vi "dataqsdk2008.vi"() -> ()   [LabVIEW 2019]
panel:
  out "Chan2":dbl(slide) scale=0.0..100.0
  out "Chan1":dbl(slide) scale=0.0..100.0
  in  "SampleRate":dbl=10.0
  in  "DeviceDriver":string="DI350NT.DLL"
  out "Two K-type inputs":dbl[][](graph)
  out "Channel 2 (K type)":dbl(knob) scale=-200.0..1372.0
  out "Channel 1 (K type)":dbl(knob) scale=-200.0..1372.0
  in  "DataqSdk":refnum<k7>(container)
  in  "Start/Stop":bool
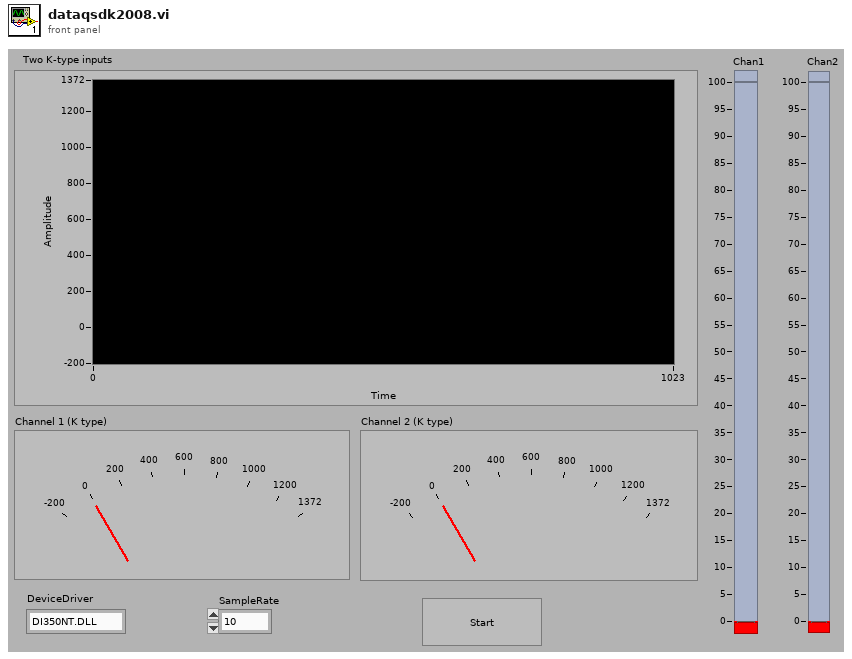
[diagram p1: front panel]
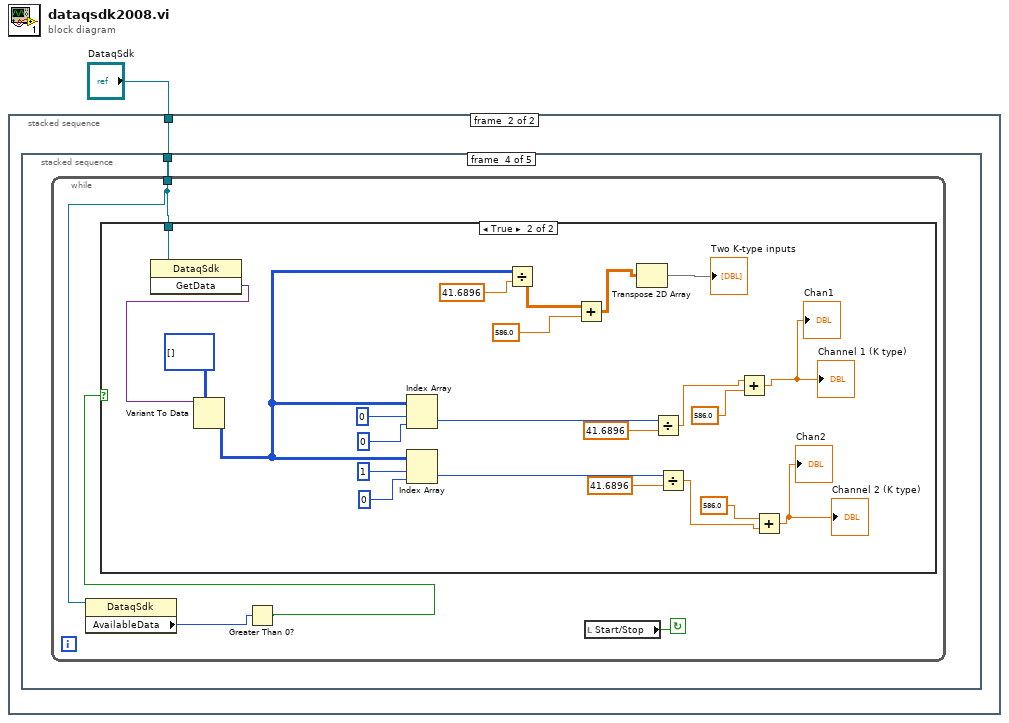
[diagram p0: block diagram]
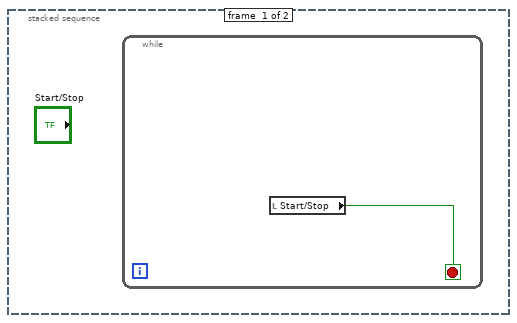
[diagram p2: hidden frame]
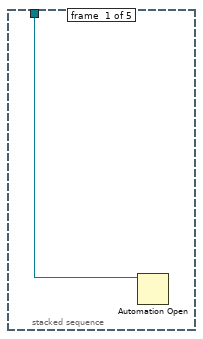
[diagram p3: hidden frame]
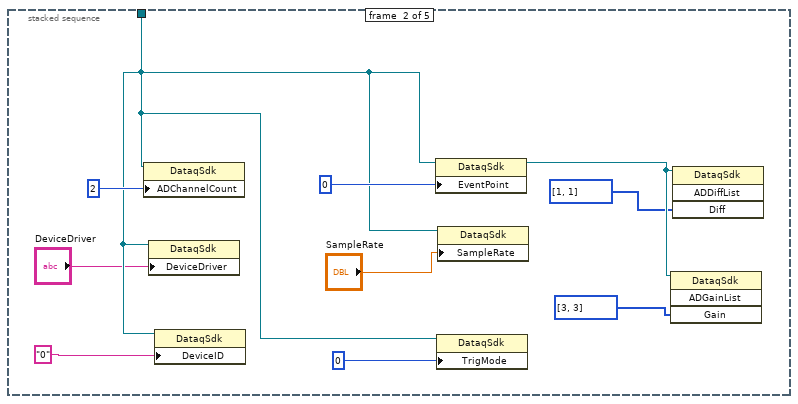
[diagram p4: hidden frame]
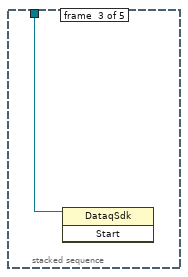
[diagram p5: hidden frame]
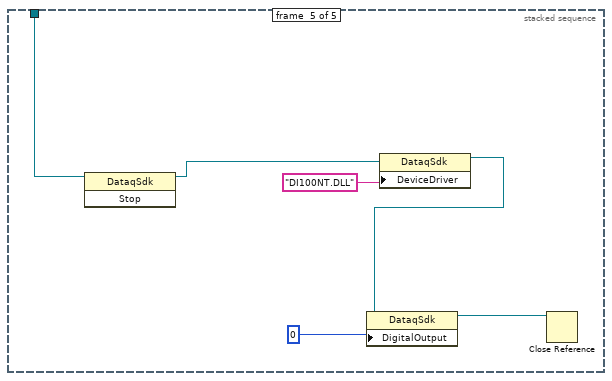
[diagram p7: hidden frame]
diagram:
  n1 = stacked-sequence {
    tunnel: "DataqSdk" -> [_ w3]
    frame #0 {
      n2 = while {
        stop <- w2 stop-if-true
        n3 = local read "Start/Stop"() -> (w2:bool)
      }
    }
    frame #1 {
      n4 = stacked-sequence {
        tunnel: w3 -> [w4 w12 w15 w16 w49]
        frame #0 {
          n5 = Automation Open(Automation Refnum=w4) -> ()  [unwired: 3 in, 2 out]
        }
        frame #1 {
          n6 = property class="DataqSdk"(reference=w12, "ADChannelCount"=2) -> ()  [unwired: 1 in, 2 out]
          n7 = property class="DataqSdk"(reference=w12, "DeviceDriver"="DeviceDriver") -> ()  [unwired: 1 in, 2 out]
          n8 = property class="DataqSdk"(reference=w12, "DeviceID"="0") -> ()  [unwired: 1 in, 2 out]
          n9 = property class="DataqSdk"(reference=w12, "EventPoint"=0) -> (reference out=w7:refnum<k7>)  [unwired: 1 in, 1 out]
          n10 = property class="DataqSdk"(reference=w12, "TrigMode"=0) -> ()  [unwired: 1 in, 2 out]
          n11 = property class="DataqSdk"(reference=w12, "SampleRate"="SampleRate") -> ()  [unwired: 1 in, 2 out]
          n12 = invoke class="DataqSdk" method="ADGainList"(reference=w7, "Gain"=i32[] [3, 3] ("Array")) -> ()  [unwired: 2 in, 4 out]
          n13 = invoke class="DataqSdk" method="ADDiffList"(reference=w7, "Diff"=i32[] [1, 1] ("Array")) -> ()  [unwired: 2 in, 4 out]
        }
        frame #2 {
          n14 = invoke class="DataqSdk" method="Start"(reference=w15) -> ()  [unwired: 2 in, 3 out]
        }
        frame #3 {
          n15 = while {
            tunnel: w16 -> [w19]
            stop <- w20 continue-if-true
            n16 = property class="DataqSdk"(reference=w19) -> ("AvailableData"=w18:i32)  [unwired: 1 in, 2 out]
            n17 = Greater Than 0?(x=w18) -> (x > 0?=w17:bool)
            n18 = case shown="True" w17 {
              tunnel: w19 -> [_ w43]
              frame False {
              }
              frame True {
                n19 = invoke class="DataqSdk" method="GetData"(reference=w43) -> ("GetData"=w39:variant)  [unwired: 2 in, 2 out]
                n20 = Variant To Data(type=i16[][] [], Variant=w39) -> (data=w32:i16[][])  [unwired: 1 in, 1 out]
                n21 = Index Array(array=w32, index (row)=0, index (col)=0) -> (element=w31:i16)
                n22 = Index Array(array=w32, index (row)=1, index (col)=0) -> (element=w30:i16)
                n23 = Divide(x=w32, y=41.6896) -> (x/y=w29:dbl[][])
                n24 = Add(x=w29, y=586.0) -> (x+y=w28:dbl[][])
                n25 = Transpose 2D Array(2D array=w28) -> (transposed array=→"Two K-type inputs":dbl[][])
                n26 = Divide(x=w31, y=41.6896) -> (x/y=w25:dbl)
                n27 = Divide(x=w30, y=41.6896) -> (x/y=w26:dbl)
                n28 = Add(x=w25, y=586.0) -> (x+y=→"Channel 1 (K type)" →"Chan1":dbl)
                n29 = Add(x=586.0, y=w26) -> (x+y=→"Channel 2 (K type)" →"Chan2":dbl)
              }
            }
            n30 = local read "Start/Stop"() -> (w20:bool)
          }
        }
        frame #4 {
          n31 = invoke class="DataqSdk" method="Stop"(reference=w49) -> (reference out=w48:refnum<k7>)  [unwired: 2 in, 2 out]
          n32 = property class="DataqSdk"(reference=w48, "DeviceDriver"="DI100NT.DLL") -> (reference out=w47:refnum<k7>)  [unwired: 1 in, 1 out]
          n33 = property class="DataqSdk"(reference=w47, "DigitalOutput"=0) -> (reference out=w46:refnum<k7>)  [unwired: 1 in, 1 out]
          n34 = Close Reference(reference=w46) -> ()  [unwired: 1 in, 1 out]
        }
      }
    }
  }
